vi "Create Station.vi"(8 "error in (no error)":errorcluster, 11 "PLC Sim Controller Actor in":refnum<class "PLC Sim Controller Actor.lvclass">) -> (0 "error out":errorcluster, 3 "PLC Sim Controller Actor out":refnum<class "PLC Sim Controller Actor.lvclass">)   [LabVIEW 2019, in "PLC Sim Controller Actor.lvlib" / "PLC Sim Controller Actor.lvclass"]
uses:
  PLC Sim Controller Actor.lvclass
  C:/Program Files (x86)/National Instruments/LabVIEW 2019/vi.lib/ActorFramework/Actor/Actor.lvclass
  Station Actor/Station Actor/Station Actor.lvclass
  <vilib>/OPCUA/controls/OPC UA Server Refnum.ctl
  PLC Sim Controller Actor.lvclass/PLC Sim Controller Actor.ctl
  Station Actor/Station Actor Messages/Set Window Title Msg/Set Window Title Msg.lvclass/Set Window Title Msg.ctl
  <vilib>/ActorFramework/Message Enqueuer/Message Enqueuer.lvclass/Message Enqueuer.ctl
  Station Actor/Station Actor Messages/Set TagIDs Msg/Set TagIDs Msg.lvclass/Set TagIDs Msg.ctl
  <vilib>/ActorFramework/Message Enqueuer/Enqueue.vi
  Station Actor/Station Actor Messages/Set Window Title Msg/Set Window Title Msg.lvclass
  C:/Program Files (x86)/National Instruments/LabVIEW 2019/vi.lib/ActorFramework/Message/Message.lvclass
  Station Actor/Station Actor Messages/Set TagIDs Msg/Set TagIDs Msg.lvclass
  <vilib>/ActorFramework/Message Priority Queue/Priority Enqueue.vi
  <vilib>/ActorFramework/Actor/Actor.lvclass
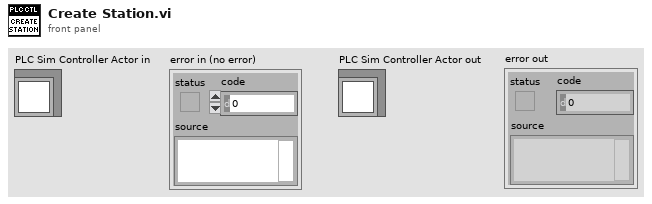
[diagram p1: front panel]
types:
  T1 = typedef "OPC UA Server Refnum.ctl" = refnum<k21>
  T2 = cluster{"OPC UA server":T1, "Rx Folder NodeID":string, "Tx Folder NodeID":string}
  T3 = map{string, refnum<class "Message Enqueuer.lvclass">}
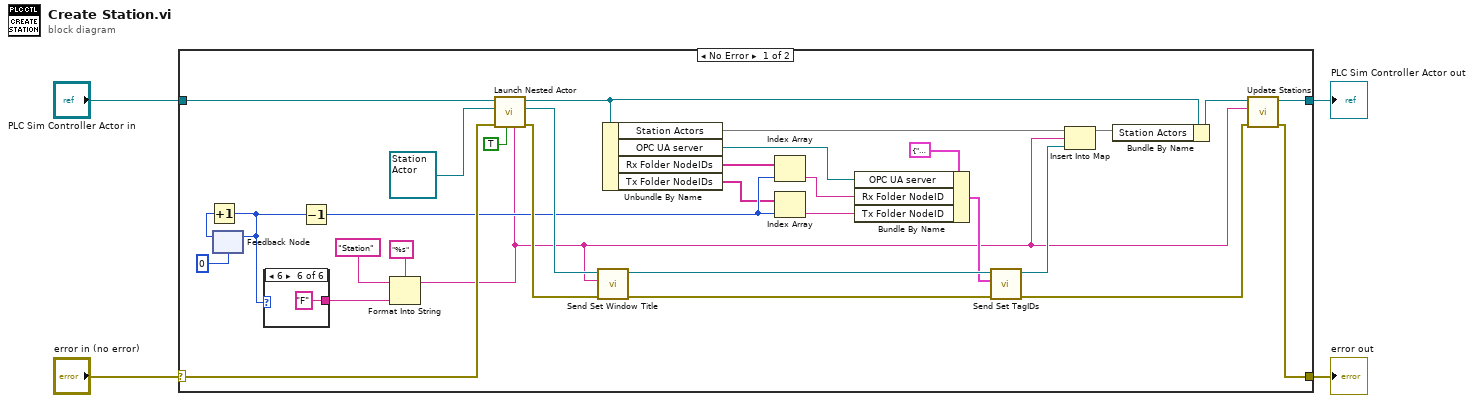
[diagram p0: block diagram]
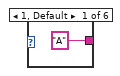
[diagram p2: hidden frame]
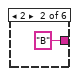
[diagram p3: hidden frame]
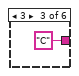
[diagram p4: hidden frame]
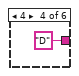
[diagram p5: hidden frame]
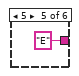
[diagram p6: hidden frame]
diagram:
  n1 = case shown="No Error" "error in (no error)" {
    selector: "error in (no error)" -> [w34 w43]
    tunnel: [w28 w43] -> w3
    tunnel: [w29 w42] -> w1
    tunnel: "PLC Sim Controller Actor in" -> [w25 w42]
    frame No Error {
      n2 = feedback #1(0) -> (w24:i32)
      n3 = Increment(x=w24) -> (x+1=w23:i32)
      n4 = feedback-in #1(w23) -> ()
      n5 = case shown="6" w23 {
        tunnel: ["A" "B" "C" "D" "E" "F"] -> w31
        frame 1, Default {
        }
        frame 2 {
        }
        frame 3 {
        }
        frame 4 {
        }
        frame 5 {
        }
        frame 6 {
        }
      }
      n6 = Decrement(x=w23) -> (x-1=w14:i32)
      n7 = Format Into String(format string="%s", initial string="Station", w31) -> (resulting string=w5:string)  [unwired: 1 in, 1 out]
      n8 = call <vilib>:"Launch Nested Actor.vi"("Debug Alias"=w5, "Open Actor Core front panel? (F)"=TRUE, "error in (no error)"=w34, "Nested Actor"=refnum<class "Station Actor.lvclass"> refnum ("Station Actor.lvlib:Station Actor.lvclass"), "Caller Actor in"=w25) -> ("error out"=w19:errorcluster, "Nested Actor's Enqueuer"=w26:refnum<class "Message Enqueuer.lvclass">, "Caller Actor out"=w21:refnum<class "PLC Sim Controller Actor.lvclass">)  [unwired: 4 in]
      n9 = call "Send Set Window Title.vi"("error in (no error)"=w19, "FP Window:Title"=w5, "Message Enqueuer"=w26) -> ("error out"=w9:errorcluster, "Message Enqueuer out"=w10:refnum<class "Message Enqueuer.lvclass">)  [unwired: 7 in]
      n10 = Unbundle By Name(w21) -> ("Station Actors"=w22:T3, "OPC UA server"=w17:T1, "Rx Folder NodeIDs"=w16:string[], "Tx Folder NodeIDs"=w13:string[])
      n11 = Index Array(array=w16, index=w14) -> (element=w15:string)
      n12 = Index Array(array=w13, index=w14) -> (element=w12:string)
      n13 = Bundle By Name(cluster=T2 {"OPC UA server"="", "Rx Folder NodeID"="", "Tx Folder NodeID"=""}, "OPC UA server"=w17, "Rx Folder NodeID"=w15, "Tx Folder NodeID"=w12) -> (w8:T2)
      n14 = call "Send Set TagIDs.vi"("error in (no error)"=w9, "Folder Info"=w8, "Message Enqueuer"=w10) -> ("error out"=w6:errorcluster, "Message Enqueuer out"=w7:refnum<class "Message Enqueuer.lvclass">)  [unwired: 7 in]
      n15 = Insert Into Map(map in=w22, key=w5, value=w7) -> (map out=w20:T3)  [unwired: 2 out]
      n16 = Bundle By Name(cluster=w21, "Station Actors"=w20) -> (w11:refnum<class "PLC Sim Controller Actor.lvclass">)
      n17 = call "Update Stations.vi"("error in (no error)"=w6, "Combo Value"=w5, "OPC Server in"=w11) -> ("error out"=w28:errorcluster, "OPC Server out"=w29:refnum<class "PLC Sim Controller Actor.lvclass">)  [unwired: 7 in]
    }
    frame Error {
    }
  }
  "error out" <- w3
  "PLC Sim Controller Actor out" <- w1
